vi "Hellicopter Controlller.vi"(0 "ElevRef":dbl, 1 "Model Parameters":T4 {"DT KF State-Space Model"."Transport Delay" format="%.2f"; "DT KF State-Space Model"."D" format="%#.2g"; "DT KF State-Space Model"."C" format="%#.2g"; "DT KF State-Space Model"."B" format="%#.2g"; "DT KF State-Space Model"."A" format="%#.2g"; "DT KF State-Space Model"."properties"."Sampling Time" format="%#.6p"; "DT KF State-Space Model"."properties"."Output Delays" format="%.4f"; "DT KF State-Space Model"."properties"."Input Delays" format="%.4f"}, 5 "ElevFB":dbl, 7 "TravRef":dbl, 9 "TravFB":dbl, 11 "Error In":errorcluster, 12 "PitchFB":dbl) -> (4 "Fan Control (Raw)":dbl[](array[numeric]), 6 "Fan Control (Bounded)":dbl[](array[numeric]), 8 "KF Output":dbl[](array[numeric]), 10 "state x(k)":dbl[](array[numeric]), 15 "Error Out":errorcluster)   [LabVIEW 2017]
uses:
  <vilib>/Analysis/Matrix/Datatypes/RealMatrix.ctl
  <vilib>/addons/Control Design/_Model Construction/Model Typedefs.llb/CD State Space Model (MIMO).ctl
  <vilib>/addons/Control Design/_Model Construction/Model Typedefs.llb/CD General Elements.ctl
  <vilib>/Simulation/DiscreteLinear/Implementation/NILVSim Discrete State Space Direct.llb/SIM Discrete State Space Direct Diagram (CD).vi
  <vilib>/Analysis/baseanly.llb/A x Vector.vi
  <vilib>/Simulation/DiscreteLinear/Implementation/Shared/SIM Init Discrete States.vi
  <vilib>/Simulation/DiscreteLinear/Implementation/NILVSim Discrete State Space Direct.llb/NILVSim Discrete State Space Direct Diagram Core (MIMO).vi
  <vilib>/Simulation/Implementation/Shared/SIM BuildSimErr.vi
  <vilib>/Simulation/Implementation/XNodeFramework/SimXNode/SimX.xnode
  <vilib>/Analysis/NI_AALBase.lvlib
  <vilib>/addons/Control Design/_Model Construction/NI_LinSys_Model Typedefs.lvlib
  <vilib>/Analysis/Matrix/NI_Matrix.lvlib
panel:
  out "state x(k+1)":dbl[](array[numeric])
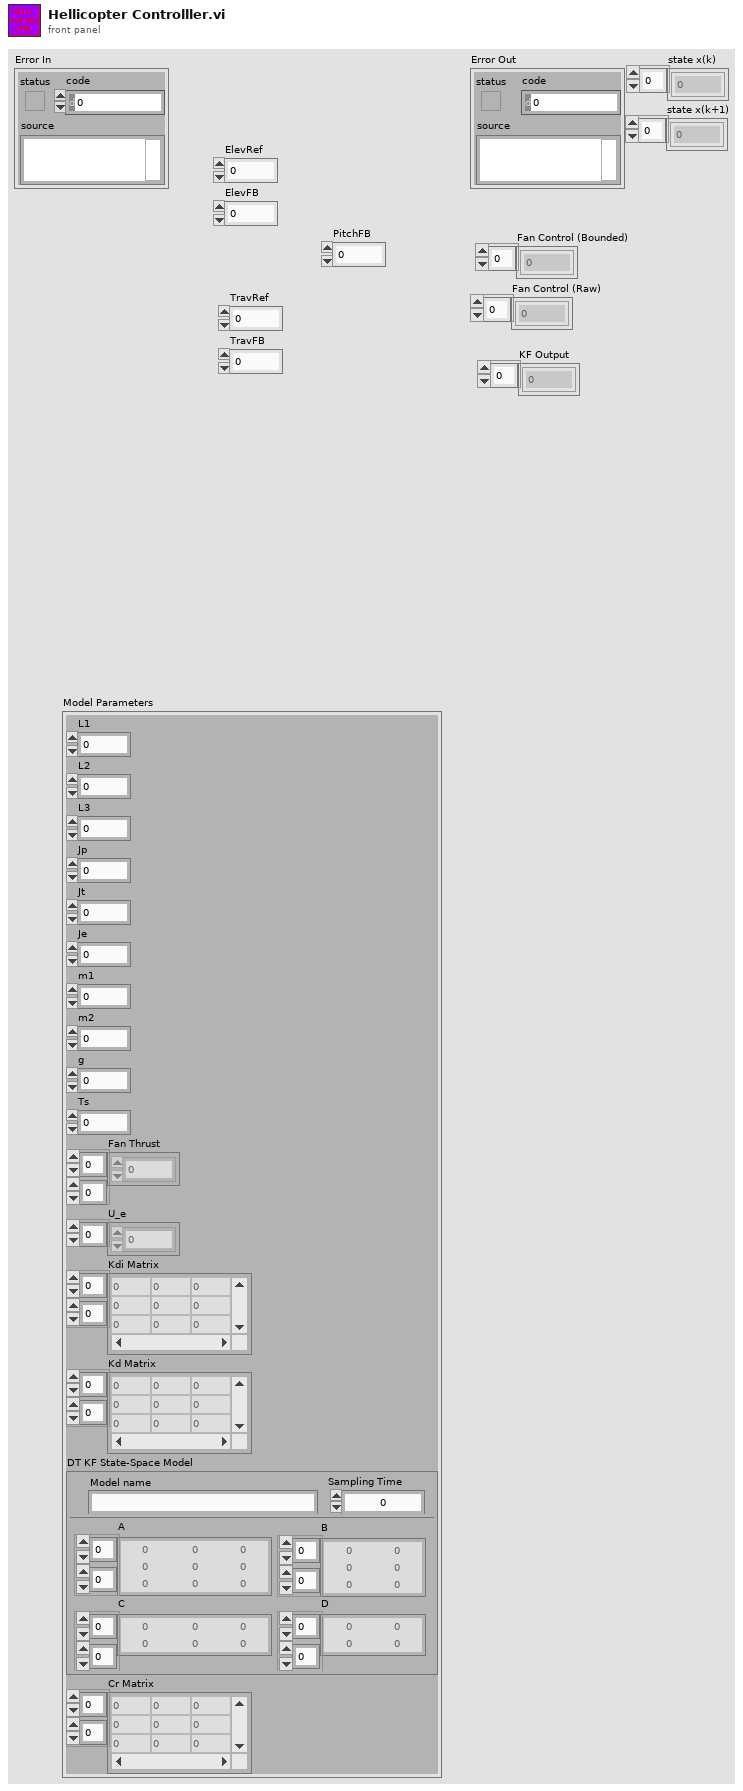
[diagram p1: front panel]
types:
  T1 = typedef "NI_Matrix.lvlib/RealMatrix.ctl" = dbl[][]
  T2 = typedef "NI_LinSys_Model Typedefs.lvlib/CD State Space Model (MIMO).ctl" = cluster{"properties":T3, "A":dbl[][], "B":dbl[][], "C":dbl[][], "D":dbl[][], "StateNames":string[], "Transport Delay":dbl[][]}
  T3 = typedef "NI_LinSys_Model Typedefs.lvlib/CD General Elements.ctl" = cluster{"Model name":string, "Input names":string[], "Output names":string[], "Input Delays":dbl[], "Output Delays":dbl[], "Sampling Time":dbl, "Notes":string}
  T4 = cluster{"L1":dbl, "L2":dbl, "L3":dbl, "Jp":dbl, "Jt":dbl, "Je":dbl, "m1":dbl, "m2":dbl, "g":dbl, "Ts":dbl, "Fan Thrust":dbl[][], "U_e":dbl[], "Kdi Matrix":T1, "Kd Matrix":T1, "DT KF State-Space Model":T2, "Cr Matrix":T1}
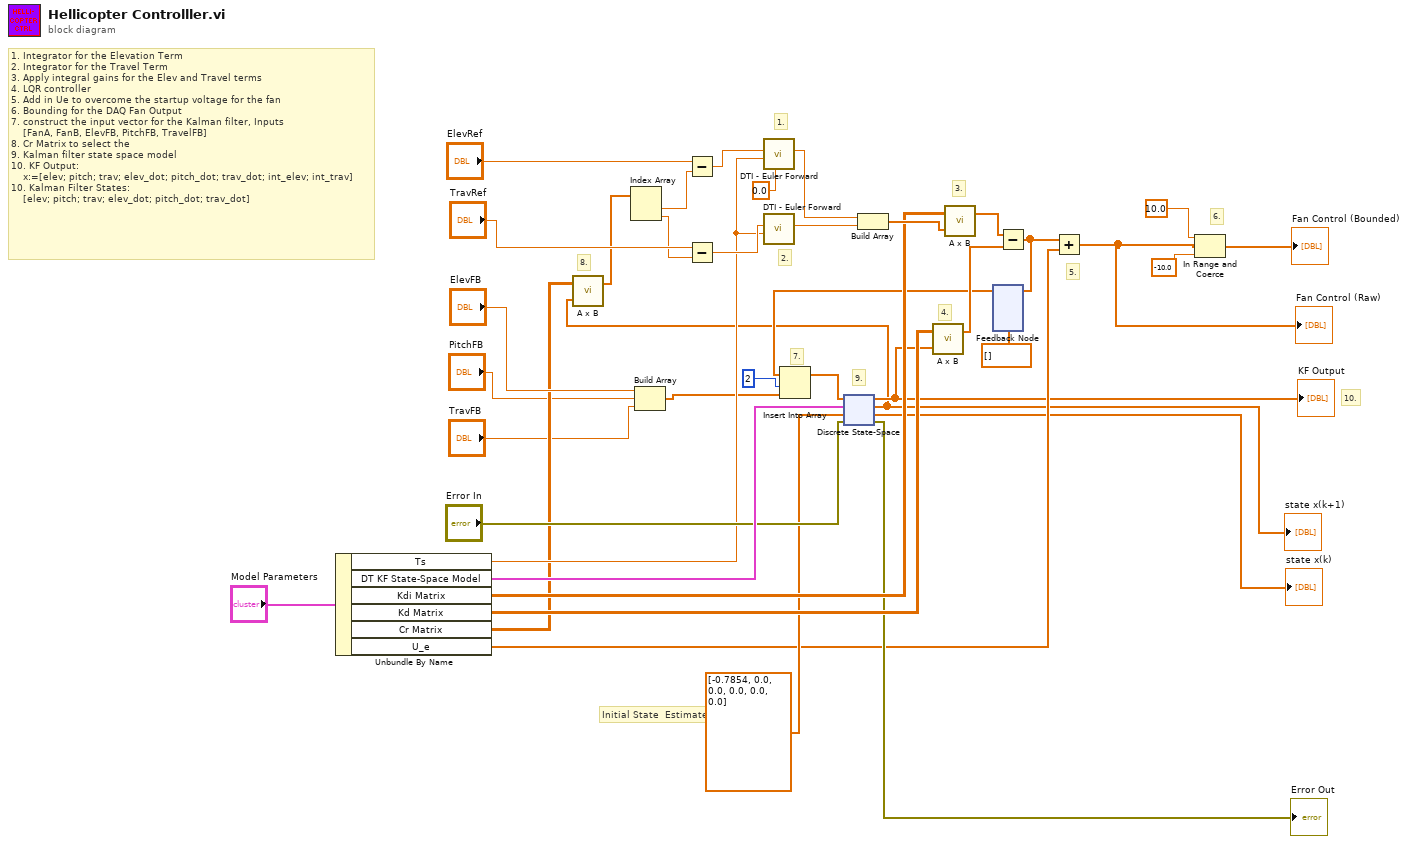
[diagram p0: block diagram]
diagram:
  # "10."
  # "1. Integrator for the Elevation Term\n2. Integrator for the Travel Term\n3. Apply integral gains for the Elev and Travel terms\n4. LQR controller\n5. Add in Ue to overcome the startup voltage for the fan\n6. Bounding for the DAQ Fan Output\n7. construct the input vector for the Kalman filter, Inputs\n    [FanA, FanB, ElevFB, PitchFB, TravelFB]\n8. Cr Matrix to select the \n9. Kalman filter state space model\n10. KF Output:\n    x:=[elev; pitch; trav; elev_dot; pitch_dot; trav_dot; int_elev; int_trav]\n10. Kalman Filter States:\n    [elev; pitch; trav; elev_dot; pitch_dot; trav_dot]"
  # "9."
  # "8."
  # "7."
  # "6."
  # "5."
  # "4."
  # "3."
  # "2."
  # "1."
  # "Initial State  Estimates"
  n1 = Unbundle By Name("Model Parameters") -> ("Ts"=w24:dbl, "DT KF State-Space Model"=w30:T2, "Kdi Matrix"=w32:T1, "Kd Matrix"=w31:T1, "Cr Matrix"=w8:T1, "U_e"=w10:dbl[])
  n2 = Build Array("ElevFB", "PitchFB", "TravFB") -> (w14:dbl[])
  n3 = feedback #1(dbl[] []) -> (w15:dbl[])
  n4 = Insert Into Array(array=w15, index=2, new element=w14) -> (w16:dbl[])
  n5 = xnode ("Discrete State-Space")("input u(k)"=w16, "State-Space"=w30, "initial state (x0)"=dbl[] [-0.7854, 0.0, 0.0, 0.0, 0.0, 0.0], "error in (no error)"="Error In") -> ("state x(k+1)"=w4:dbl[], "output y(k)"=w7:dbl[], "state x(k)"=→"state x(k)":dbl[], "error out"=→"Error Out":errorcluster)  [unwired: 1 in]
  "KF Output" <- w7
  "state x(k+1)" <- w4
  n6 = call-poly <vilib>:"A x B.vi"("Vector"=w4, "A"=w8) -> ("A x Vector"=w6:dbl[])  [unwired: 1 out]
  n7 = Index Array(array=w6) -> (element #1=w9:dbl, element #2=w1:dbl)  [unwired: 2 in]
  n8 = Subtract(x="ElevRef", y=w9) -> (x-y=w23:dbl)
  n9 = Subtract(x="TravRef", y=w1) -> (x-y=w26:dbl)
  n10 = call "DTI - Euler Forward.vi"("Init"=0.0, "Ts"=w24, "U"=w23) -> ("Y"=w22:dbl)  [unwired: 8 in]
  n11 = call "DTI - Euler Forward.vi"("Ts"=w24, "U"=w26) -> ("Y"=w25:dbl)  [unwired: 9 in]
  n12 = Build Array(w22, w25) -> (w37:dbl[])
  n13 = call-poly <vilib>:"A x B.vi"("Vector"=w7, "A"=w31) -> ("A x Vector"=w38:dbl[])  [unwired: 1 out]
  n14 = call-poly <vilib>:"A x B.vi"("Vector"=w37, "A"=w32) -> ("A x Vector"=w39:dbl[])  [unwired: 1 out]
  n15 = Subtract ("Subtract.vi")(x=w39, y=w38) -> (x-y=w29:dbl[])
  n16 = feedback-in #1(w29) -> ()
  n17 = Add(x=w29, y=w10) -> (x+y=w18:dbl[])
  "Fan Control (Raw)" <- w18
  n18 = In Range and Coerce(upper limit=10.0, x=w18, lower limit=-10.0) -> (coerced(x)=→"Fan Control (Bounded)":dbl[])  [unwired: 1 out]
